vi "Create Pattern Script(one timeset).vi"(7 "Notes":string, 9 "PinState":enum16{"0", "1", "L", "H", "X", "V", "D", "M"}[](array[ring]), 10 "timeset name":string="-", 11 "opcode":string) -> (3 "string out":string)   [LabVIEW 2018, in "BML_Frame_Root.lvclass"]
uses:
  BML_Frame_Root.lvclass
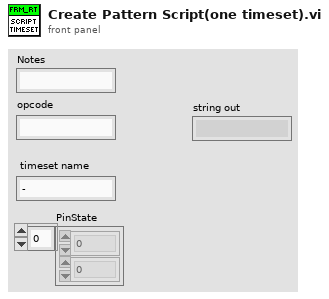
[diagram p1: front panel]
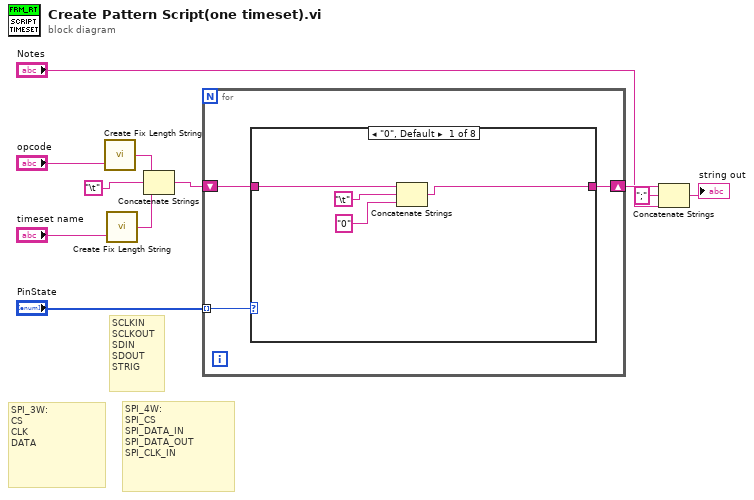
[diagram p0: block diagram]
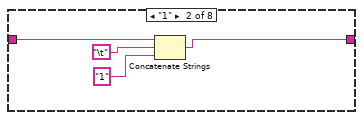
[diagram p2: hidden frame]
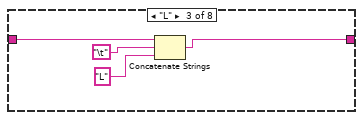
[diagram p3: hidden frame]
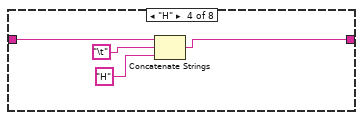
[diagram p4: hidden frame]
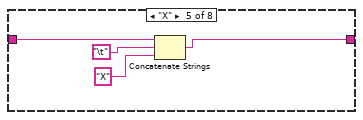
[diagram p5: hidden frame]
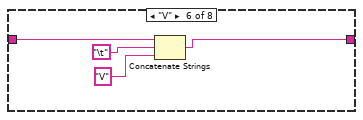
[diagram p6: hidden frame]
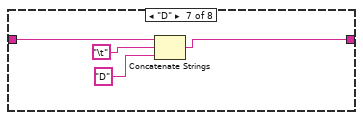
[diagram p7: hidden frame]
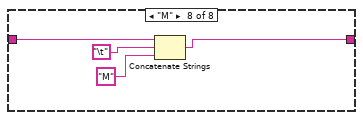
[diagram p8: hidden frame]
diagram:
  # "SPI_3W:\nCS\nCLK\nDATA"
  # "SPI_4W:\nSPI_CS\nSPI_DATA_IN\nSPI_DATA_OUT\nSPI_CLK_IN"
  # "SCLKIN\nSCLKOUT\nSDIN\nSDOUT\nSTRIG"
  n1 = call "Create Fix Length String.vi"("String"="opcode") -> ("String out"=w4:string)  [unwired: 1 in]
  n2 = call "Create Fix Length String.vi"("String"="timeset name") -> ("String out"=w2:string)  [unwired: 1 in]
  n3 = Concatenate Strings(w4, "\t", w2) -> (w9:string)
  n4 = for {
    tunnel: "PinState" -> [w14] mode=indexing
    shift-right: [w12] -> w8
    shift-left: w9 -> [w13]
    n5 = case shown="\"0\", Default" w14 {
      tunnel: w13 -> [w18 w22 w26 w30 w34 w38 w42 w46]
      tunnel: [w15 w19 w23 w27 w31 w35 w39 w43] -> w12
      frame "0", Default {
        n6 = Concatenate Strings(w18, "\t", "0") -> (w15:string)
      }
      frame "1" {
        n7 = Concatenate Strings(w22, "\t", "1") -> (w19:string)
      }
      frame "L" {
        n8 = Concatenate Strings(w26, "\t", "L") -> (w23:string)
      }
      frame "H" {
        n9 = Concatenate Strings(w30, "\t", "H") -> (w27:string)
      }
      frame "X" {
        n10 = Concatenate Strings(w34, "\t", "X") -> (w31:string)
      }
      frame "V" {
        n11 = Concatenate Strings(w38, "\t", "V") -> (w35:string)
      }
      frame "D" {
        n12 = Concatenate Strings(w42, "\t", "D") -> (w39:string)
      }
      frame "M" {
        n13 = Concatenate Strings(w46, "\t", "M") -> (w43:string)
      }
    }
  }
  n14 = Concatenate Strings(w8, ";" ("string"), "Notes") -> (→"string out":string)
